vi "Generate New File.vi"(8 "error in":errorcluster, 11 "File Actor in":refnum<class "File Actor.lvclass">) -> (0 "error out":errorcluster, 3 "File Actor out":refnum<class "File Actor.lvclass">)   [LabVIEW 2018, in "File Library.lvlib" / "File Actor.lvclass"]
doc: "Open a new file using the current configuration parameters stored in the object. If a file is currently open, close it. If there is a header, write it to the file.\n\nThe file reference itself is written to a DVR - this allows the sharing of the refreence across multiple loops (as in the File::Actor Core)."
uses:
  File Actor.lvclass
  C:/Users/Labview/Documents/exscalabar_server/SuperActor/SuperActor.lvclass
  File Actor.lvclass/File Actor.ctl
  SuperActor/SuperActor.lvclass/SuperActor.ctl
  SuperActor/Read Log Session.vi
  <userlib>/_Session Fwk/Session - Root.lvclass
  reusable/Session APIs/Session Log/System Log.lvclass
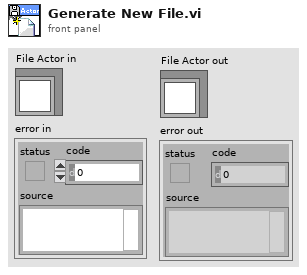
[diagram p1: front panel]
types:
  T1 = enum16{"open", "replace", "create", "open or create", "replace or create", "replace or create with confirmation"}
  T2 = typedef "Session - Root.lvclass/Session Handle.ctl" = refnum<data-value>
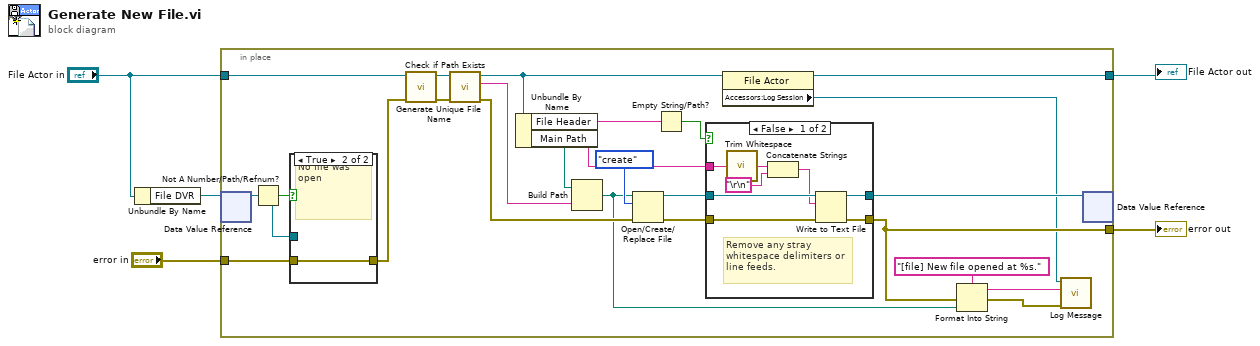
[diagram p0: block diagram]
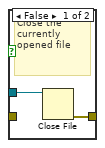
[diagram p3: hidden frame]
diagram:
  n1 = Unbundle By Name("File Actor in") -> ("File DVR"=w5:refnum<data-value>)
  n2 = in-place {
    in-place-border: "File Actor in" -> [w15]
    in-place-border: [w7] -> w2
    in-place-border: [w11] -> w3
    in-place-border: "error in" -> [w6]
    n3 = in-place-dvr #1(w5) -> (w17:refnum<file>)  [unwired: 1 out]
    n4 = Not A Number/Path/Refnum?(number/path/refnum=w17) -> (NaN/Path/Refnum?=w28:bool)
    n5 = case shown="True" w28 {
      tunnel: [w41 w42] -> w12
      tunnel: w17 -> [w40 _]
      tunnel: w6 -> [_ w42]
      frame False {
        # "Close the currently opened file"
        n6 = Close File(refnum=w40) -> (error out=w41:errorcluster)  [unwired: 1 in, 1 out]
      }
      frame True {
        # "No file was open"
      }
    }
    n7 = call "Check if Path Exists.vi"("error in"=w12, "File Actor in"=w15) -> ("error out"=w13:errorcluster, "File Actor out"=w14:refnum<class "File Actor.lvclass">)  [unwired: 8 in]
    n8 = call "Generate Unique File Name.vi"("error in"=w13, "File Actor in"=w14) -> ("error out"=w22:errorcluster, "File Name"=w27:string, "File Actor out"=w9:refnum<class "File Actor.lvclass">)  [unwired: 7 in]
    n9 = Unbundle By Name(w9) -> ("File Header"=w23:string, "Main Path"=w16:path)
    n10 = Build Path(base path=w16, name or relative path=w27) -> (appended path=w21:path)
    n11 = Open/Create/Replace File(file path (use dialog)=w21, error in=w22, operation (0:open)=T1."create") -> (refnum out=w25:refnum<file>, error out=w24:errorcluster)  [unwired: 4 out]
    n12 = Empty String/Path?(string/path=w23) -> (empty?=w26:bool)
    n13 = case shown="False" w26 {
      tunnel: w25 -> [w37 w39]
      tunnel: w24 -> [w36 w38]
      tunnel: [w35 w39] -> w18
      tunnel: [w34 w38] -> w11
      tunnel: w23 -> [w31 _]
      frame False {
        # "Remove any stray whitespace delimiters or line feeds."
        n14 = call <vilib>:"Trim Whitespace.vi"("string"=w31) -> ("trimmed string"=w30:string)  [unwired: 1 in]
        n15 = Concatenate Strings(w30, "\r\n") -> (w32:string)
        n16 = Write to Text File(file (use dialog)=w37, text=w32, error in=w36) -> (refnum out=w35:refnum<file>, error out=w34:errorcluster)  [unwired: 1 in, 1 out]
      }
      frame True {
        # "No header"
      }
    }
    n17 = property class="File Actor"(reference=w9) -> (reference out=w7:refnum<class "File Actor.lvclass">, "Accessors:Log Session"=w8:T2)  [unwired: 1 in, 1 out]
    n18 = Format Into String(format string="[file] New file opened at %s.", error in=w11, w21) -> (resulting string=w19:string, error out=w10:errorcluster)  [unwired: 1 in]
    n19 = call "Log Message.vi"("error in"=w10, "MSG In"=w19, "session in"=w8) -> ()  [unwired: 7 in, 2 out]
    n20 = in-place-dvr #1(w18) -> ()  [unwired: 2 out]
  }
  "error out" <- w3
  "File Actor out" <- w2
